vi "GenMsgID.vi"(10 "error in":errorcluster) -> (2 "error out":errorcluster, 3 "MsgID":u16)   [LabVIEW 2014]
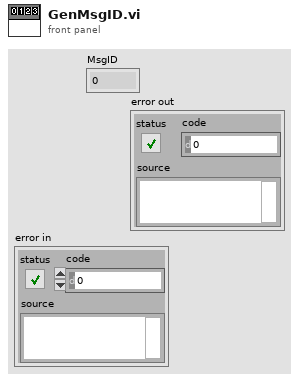
[diagram p1: front panel]
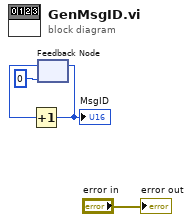
[diagram p0: block diagram]
diagram:
  n1 = feedback #1(u16 0) -> (w2:u16)
  n2 = Increment(x=w2) -> (x+1=w4:u16)
  "MsgID" <- w4
  n3 = feedback-in #1(w4) -> ()
  "error out" <- "error in"
